vi "VisionTargetRead.vi"(5 "RobotConfig":T1={"Motors"={"DriveLeftPrimary"={"CAN Address"=1, "Invert"=FALSE, "InvertSensor"=FALSE, "Unit Conversion Factor"=0.0, "Brake Mode"=enum."Override to Brake", "Reverse Limt Switch Mode"=enum."Normally Closed", "Forward Limt Swith Mode"=enum."Normally Closed"}, "DriveLeftSecondary1"={"CAN Address"=2, "Invert"=FALSE, "InvertSensor"=FALSE, "Unit Conversion Factor"=0.0, "Brake Mode"=enum."Override to Brake", "Reverse Limt Switch Mode"=enum."Normally Closed", "Forward Limt Swith Mode"=enum."Normally Closed"}, "DriveRightPrimary"={"CAN Address"=3, "Invert"=FALSE, "InvertSensor"=FALSE, "Unit Conversion Factor"=0.0, "Brake Mode"=enum."Override to Brake", "Reverse Limt Switch Mode"=enum."Normally Closed", "Forward Limt Swith Mode"=enum."Normally Closed"}, "DriveRightSecondary1"={"CAN Address"=4, "Invert"=FALSE, "InvertSensor"=FALSE, "Unit Conversion Factor"=0.0, "Brake Mode"=enum."Override to Brake", "Reverse Limt Switch Mode"=enum."Normally Closed", "Forward Limt Swith Mode"=enum."Normally Closed"}, "RightIntake"={"CAN Address"=8, "Invert"=FALSE, "InvertSensor"=FALSE, "Unit Conversion Factor"=0.0, "Brake Mode"=enum."Override to Brake", "Reverse Limt Switch Mode"=enum."Normally Closed", "Forward Limt Swith Mode"=enum."Normally Closed"}, "LeftIntake"={"CAN Address"=7, "Invert"=FALSE, "InvertSensor"=FALSE, "Unit Conversion Factor"=0.0, "Brake Mode"=enum."Override to Brake", "Reverse Limt Switch Mode"=enum."Normally Closed", "Forward Limt Swith Mode"=enum."Normally Closed"}, "ArmPivot"={"CAN Address"=5, "Invert"=FALSE, "InvertSensor"=FALSE, "Unit Conversion Factor"=0.0, "Brake Mode"=enum."Override to Brake", "Reverse Limt Switch Mode"=enum."Normally Closed", "Forward Limt Swith Mode"=enum."Normally Closed"}, "ArmExtend"={"CAN Address"=6, "Invert"=FALSE, "InvertSensor"=FALSE, "Unit Conversion Factor"=0.0, "Brake Mode"=enum."Override to Brake", "Reverse Limt Switch Mode"=enum."Normally Closed", "Forward Limt Swith Mode"=enum."Normally Closed"}, "ArmPivot2"={"CAN Address"=9, "Invert"=FALSE, "InvertSensor"=FALSE, "Unit Conversion Factor"=0.0, "Brake Mode"=enum."Override to Brake", "Reverse Limt Switch Mode"=enum."Normally Closed", "Forward Limt Swith Mode"=enum."Normally Closed"}, "Climber"={"CAN Address"=10, "Invert"=FALSE, "InvertSensor"=FALSE, "Unit Conversion Factor"=0.0, "Brake Mode"=enum."Override to Brake", "Reverse Limt Switch Mode"=enum."Disabled", "Forward Limt Swith Mode"=enum."Disabled"}}, "Sensors"={"IMU"={"Yaw Axis"=enum."Z", "SPI Bus"=enum."SPI MXP", "AHRS Algorithm"=enum."Complementary", "Calibration Time (s)"=3.0, "Calibrate On Open"=TRUE}, "LimitSwitch1"={"DIOChannel"=enum."DIO 0", "Active Low"=FALSE}, "LimitSwitch2"={"DIOChannel"=enum."DIO 1", "Active Low"=FALSE}, "BeamBreak"={"DIOChannel"=enum."DIO 2", "Active Low"=FALSE}, "JeVois"={"Baud Rate"=9600, "Parity"=0, "Data Bits"=8, "Stop Bits"=10, "Termination Char (0xA = '\\n' = LF)"=10, "Enable Termination Char? (T)"=TRUE, "Flow Control"=0, "Timeout Value (ms)"=5000, "Serial Port"=enum."Onboard RS-232"}}, "PID"={"ArmExtend"={"P"=0.0, "I"=0.0, "D"=0.0, "F"=0.0, "IZone"=0.0}, "ArmRotate"={"P"=0.0, "I"=0.0, "D"=0.0, "F"=0.0, "IZone"=0.0}, "Drive"={"P"=0.0, "I"=0.0, "D"=0.0, "F"=0.0, "IZone"=0.0}}, "Solenoids"={"ArmClaw"={"Forward Channel"=enum."Solenoid 0", "Invert"=FALSE, "Reverse Channel"=enum."Solenoid 0"}, "IntakeExtend"={"Forward Channel"=enum."Solenoid 1", "Invert"=FALSE, "Reverse Channel"=enum."Solenoid 0"}, "IntakeOpen"={"Forward Channel"=enum."Solenoid 2", "Invert"=FALSE, "Reverse Channel"=enum."Solenoid 0"}, " Shifter"={"Forward Channel"=enum."Solenoid 3", "Invert"=FALSE, "Reverse Channel"=enum."Solenoid 0"}}, "RobotDimensions "={"Length"=0.0, "Height"=0.0, "HeightOfBumpers"=0.0, "DistanceFromFrameEdgeToPyramid "=0.0, "HeightOfFrameToIntake"=0.0, "EdgeOfFrameToOrigin"=0.0}, "ArmHomePosition"={"Angle (rad)"=0.0, "Radius (in)"=0.0}} {"Sensors"."JeVois"."Flow Control" items=["None", "XON/XOFF", "RTS/CTS", "XON/XOFF & RTS/CTS", "DTR/DSR", "XON/XOFF & DTR/DSR"]; "Sensors"."JeVois"."Termination Char (0xA = '\\n' = LF)" format="%.0x"; "Sensors"."JeVois"."Stop Bits" items=["1.0"=10, "1.5"=15, "2.0"=20]; "Sensors"."JeVois"."Parity" items=["None", "Odd", "Even", "Mark", "Space"]}, 6 "JeVois Camera DevRef":T16) -> (0 "error out":errorcluster, 1 "Right Vision Target":T17, 2 "Left Vision Target":T17, 3 "JeVoisOut":T16, 4 "Power Cube":T17)   [LabVIEW 2017]
uses:
  TypeDefs/VisionTarget.ctl
  General/PathPlanning/TypeDefs/Point2D.ctl
  TypeDefs/VisionTargetType.ctl
  <vilib>/Rock Robotics/WPI/SerialPort/WPI_SerialPortRef.ctl
  TypeDefs/ConfigComponents/Config_Robot.ctl
  TypeDefs/ConfigComponents/Config_Motor.ctl
  <vilib>/Rock Robotics/WPI/ThirdParty/Phoenix-LabVIEW/Motor Controller/Controls/CTRE_Phoenix_MotorControl_NeutralMode.ctl
  <vilib>/Rock Robotics/WPI/ThirdParty/Phoenix-LabVIEW/Motor Controller/Controls/CTRE_Phoenix_MotorControl_LimitSwitchNormal.ctl
  TypeDefs/ConfigComponents/Config_IMU.ctl
  <vilib>/Rock Robotics/SystemInterfaces/spilib/spi_bus.ctl
  TypeDefs/ConfigComponents/Config_DigitalIO.ctl
  <vilib>/Rock Robotics/SystemInterfaces/DIO/FPGA_DIOChannel.ctl
  TypeDefs/ConfigComponents/Config_SerialPort.ctl
  <vilib>/Rock Robotics/WPI/SerialPort/WPI_SerialPort.ctl
  TypeDefs/ConfigComponents/Config_PIDParams.ctl
  TypeDefs/ConfigComponents/Config_DoubleSolenoid.ctl
  <vilib>/Rock Robotics/WPI/Solenoid/WPI_SolenoidChannel.ctl
  TypeDefs/ConfigComponents/Config_Dimensions.ctl
  TypeDefs/ConfigComponents/Config_ArmHome.ctl
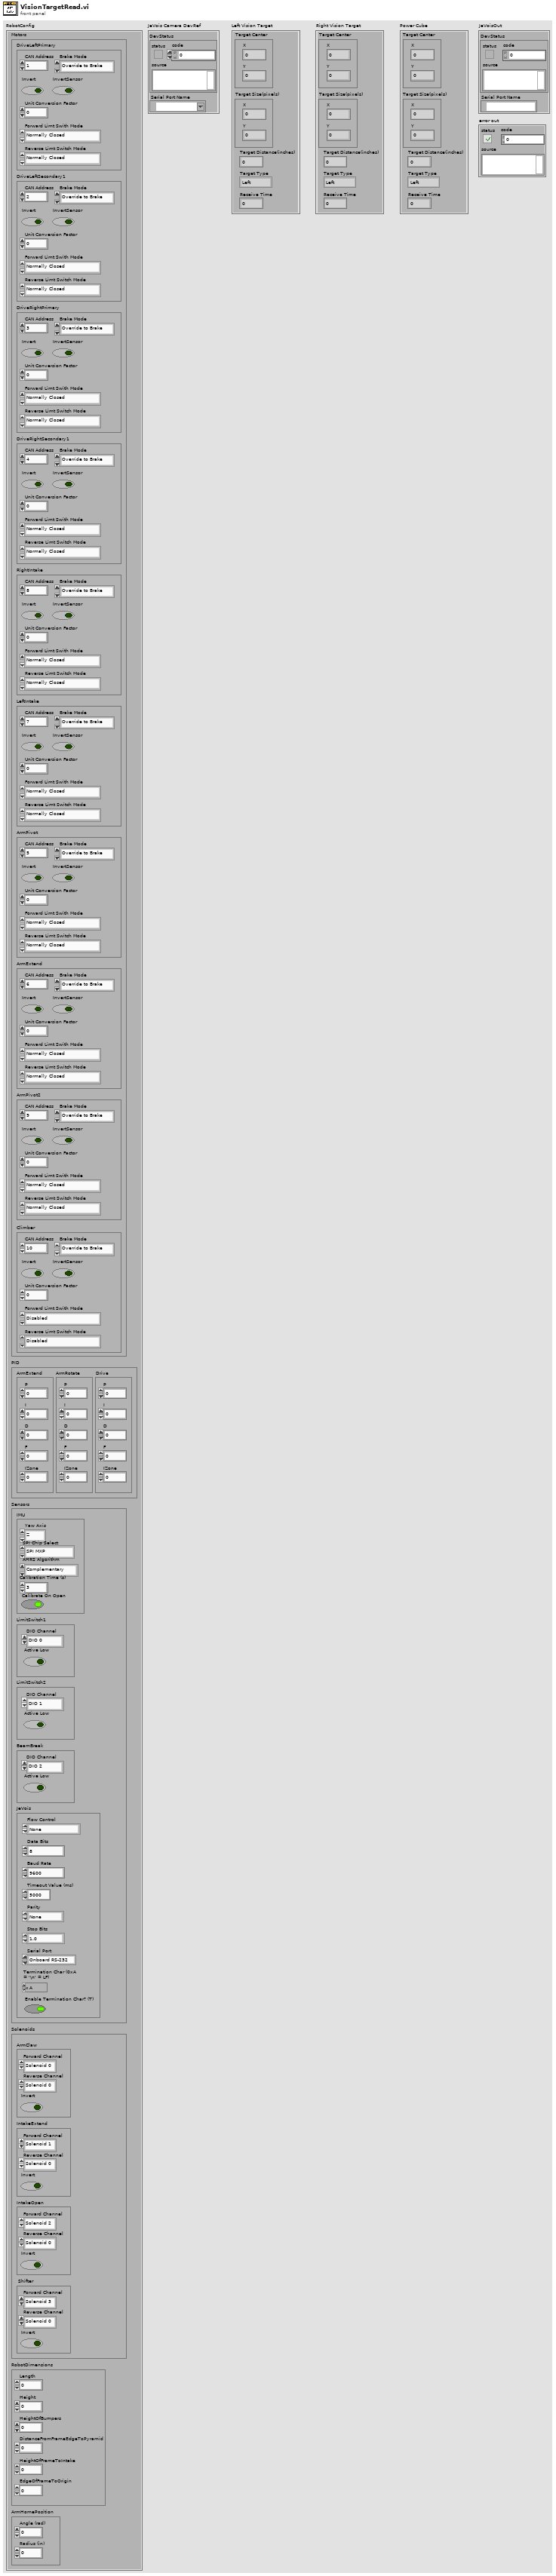
[diagram p1: front panel]
types:
  T1 = typedef "Config_Robot.ctl" = cluster{"Motors":cluster{"DriveLeftPrimary":T2, "DriveLeftSecondary1":T2, "DriveRightPrimary":T2, "DriveRightSecondary1":T2, "RightIntake":T2, "LeftIntake":T2, "ArmPivot":T2, "ArmExtend":T2, "ArmPivot2":T2, "Climber":T2}, "Sensors":cluster{"IMU":T5, "LimitSwitch1":T7, "LimitSwitch2":T7, "BeamBreak":T7, "JeVois":T9}, "PID":cluster{"ArmExtend":T11, "ArmRotate":T11, "Drive":T11}, "Solenoids":cluster{"ArmClaw":T12, "IntakeExtend":T12, "IntakeOpen":T12, " Shifter":T12}, "RobotDimensions ":T14, "ArmHomePosition":T15}
  T2 = typedef "Config_Motor.ctl" = cluster{"CAN Address":u8, "Invert":bool, "InvertSensor":bool, "Unit Conversion Factor":dbl, "Brake Mode":T3, "Reverse Limt Switch Mode":T4, "Forward Limt Swith Mode":T4}
  T3 = typedef "CTRE_Phoenix_MotorControl_NeutralMode.ctl" = enum8{"EEPROMSetting", "Override to Coast", "Override to Brake"}
  T4 = typedef "CTRE_Phoenix_MotorControl_LimitSwitchNormal.ctl" = enum16{"Normally Open", "Normally Closed", "Disabled"}
  T5 = typedef "Config_IMU.ctl" = cluster{"Yaw Axis":enum16{"X", "Y", "Z"}, "SPI Bus":T6, "AHRS Algorithm":enum16{"Complementary", "Madgwick"}, "Calibration Time (s)":dbl, "Calibrate On Open":bool}
  T6 = typedef "spi_bus.ctl" = enum16{"SPI On-Board, CS0", "SPI On-Board, CS1", "SPI On-Board, CS2", "SPI On-Board, CS3", "SPI MXP", "Invalid"}
  T7 = typedef "Config_DigitalIO.ctl" = cluster{"DIOChannel":T8, "Active Low":bool}
  T8 = typedef "FPGA_DIOChannel.ctl" = enum8{"DIO 0", "DIO 1", "DIO 2", "DIO 3", "DIO 4", "DIO 5", "DIO 6", "DIO 7", "DIO 8", "DIO 9", "DIO MXP 0", "DIO MXP 1", "DIO MXP 2", "DIO MXP 3", "DIO MXP 4", "DIO MXP 5", "DIO MXP 6", "DIO MXP 7", "DIO MXP 8", "DIO MXP 9", "DIO MXP 10", "DIO MXP 11", "DIO MXP 12", "DIO MXP 13", "DIO MXP 14", "DIO MXP 15", "SPI Port CS1", "SPI Port CS2", "SPI Port CS3", "SPI Port MISO", "SPI Port MOSI", "Invalid"}
  T9 = typedef "Config_SerialPort.ctl" = cluster{"Baud Rate":u32, "Parity":u16, "Data Bits":u16, "Stop Bits":u16, "Termination Char (0xA = '\\n' = LF)":u8, "Enable Termination Char? (T)":bool, "Flow Control":u16, "Timeout Value (ms)":u32, "Serial Port":T10}
  T10 = typedef "WPI_SerialPort.ctl" = enum16{"Onboard RS-232", "MXP TTL", "USB 1", "USB 2"}
  T11 = typedef "Config_PIDParams.ctl" = cluster{"P":dbl, "I":dbl, "D":dbl, "F":dbl, "IZone":dbl}
  T12 = typedef "Config_DoubleSolenoid.ctl" = cluster{"Forward Channel":T13, "Invert":bool, "Reverse Channel":T13}
  T13 = typedef "WPI_SolenoidChannel.ctl" = enum8{"Solenoid 0", "Solenoid 1", "Solenoid 2", "Solenoid 3", "Solenoid 4", "Solenoid 5", "Solenoid 6", "Solenoid 7", "Invalid"}
  T14 = typedef "Config_Dimensions.ctl" = cluster{"Length":dbl, "Height":dbl, "HeightOfBumpers":dbl, "DistanceFromFrameEdgeToPyramid ":dbl, "HeightOfFrameToIntake":dbl, "EdgeOfFrameToOrigin":dbl}
  T15 = typedef "Config_ArmHome.ctl" = cluster{"Angle (rad)":dbl, "Radius (in)":dbl}
  T16 = typedef "WPI_SerialPortRef.ctl" = cluster{"DevStatus":errorcluster, "Serial Port Name":refnum<visa-resource-name>}
  T17 = typedef "VisionTarget.ctl" = cluster{"Target Center":T18, "Target Size(pixels)":T18, "Target Distance(inches)":dbl, "Target Type":T19, "Receive Time":u32}
  T18 = typedef "Point2D.ctl" = cluster{"X":dbl, "Y":dbl}
  T19 = typedef "VisionTargetType.ctl" = enum16{"Left", "Right", "Cube", "Unknown"}
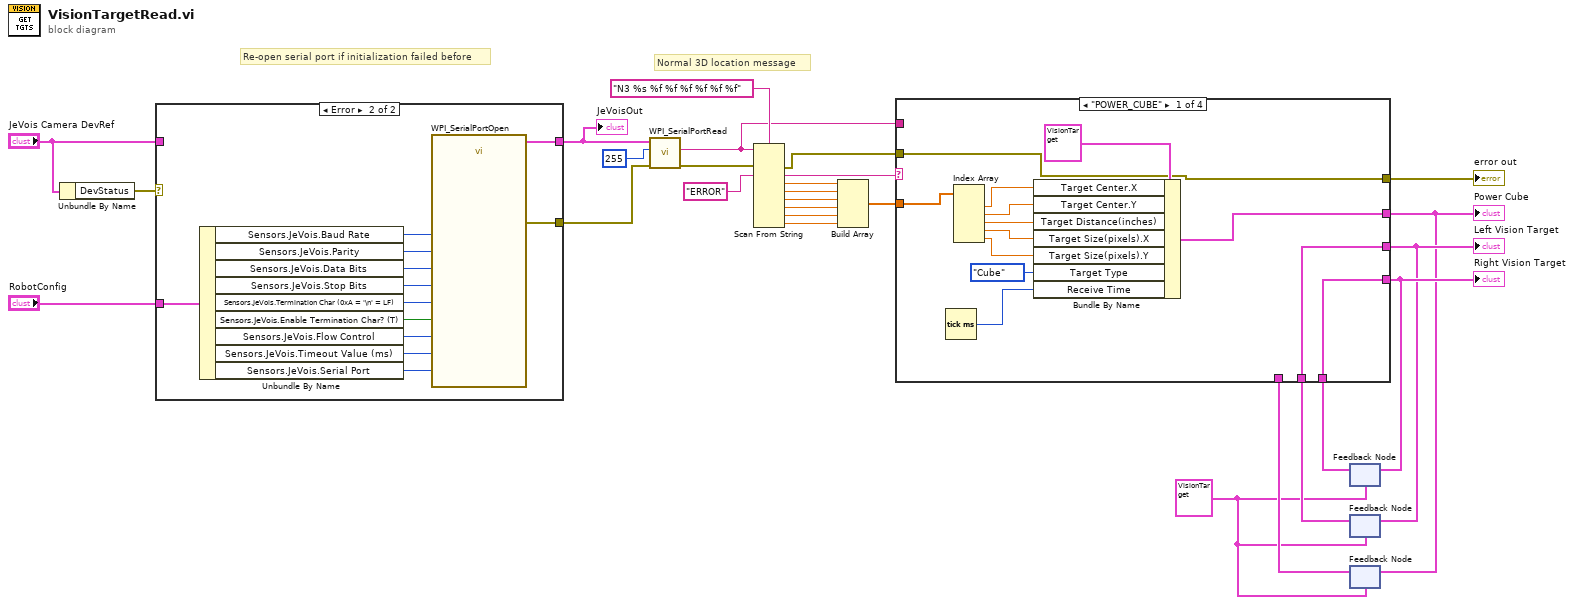
[diagram p0: block diagram]
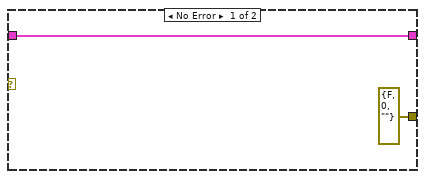
[diagram p2: hidden frame]
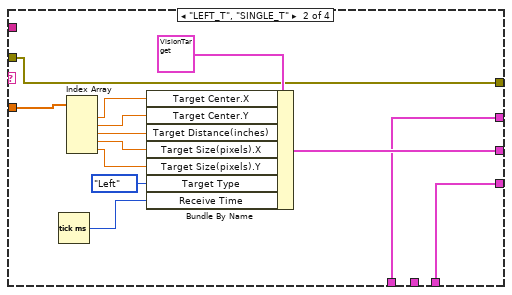
[diagram p3: hidden frame]
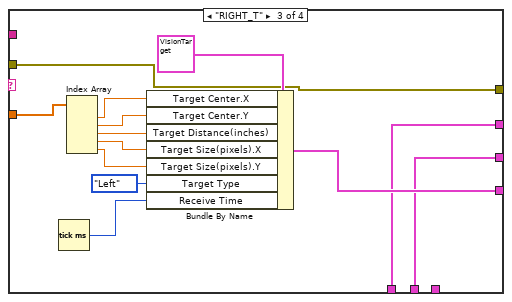
[diagram p4: hidden frame]
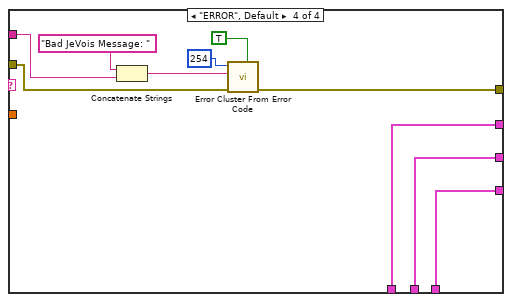
[diagram p5: hidden frame]
diagram:
  w8 = T17 {"Target Center"={"X"=0.0, "Y"=0.0}, "Target Size(pixels)"={"X"=0.0, "Y"=0.0}, "Target Distance(inches)"=0.0, "Target Type"=enum."Unknown", "Receive Time"=0} ("Left Vision Target")
  # "Re-open serial port if initialization failed before"
  # "Normal 3D location message"
  n1 = Unbundle By Name("JeVois Camera DevRef") -> ("DevStatus"=w5:errorcluster)
  n2 = case shown="Error" w5 {
    tunnel: [w29 w40] -> w3
    tunnel: "JeVois Camera DevRef" -> [w29 _]
    tunnel: [errorcluster {"status"=FALSE, "code"=0, "source"=""} ("error out") w41] -> w2
    tunnel: "RobotConfig" -> [_ w39]
    frame No Error {
    }
    frame Error {
      n3 = Unbundle By Name(w39) -> ("Sensors.JeVois.Baud Rate"=w38:u32, "Sensors.JeVois.Parity"=w37:u16, "Sensors.JeVois.Data Bits"=w36:u16, "Sensors.JeVois.Stop Bits"=w35:u16, "Sensors.JeVois.Termination Char (0xA = '\\n' = LF)"=w34:u8, "Sensors.JeVois.Enable Termination Char? (T)"=w33:bool, "Sensors.JeVois.Flow Control"=w32:u16, "Sensors.JeVois.Timeout Value (ms)"=w31:u32, "Sensors.JeVois.Serial Port"=w30:T10)
      n4 = call <vilib>:"WPI_SerialPortOpen.vi"("Baud Rate"=w38, "Timeout Value (ms)"=w31, "Termination Char (0xA = '\\n' = LF)"=w34, "Enable Termination Char? (T)"=w33, "Data Bits"=w36, "Parity"=w37, "Stop Bits"=w35, "Flow Control"=w32, "Serial Port"=w30) -> ("SerialPortRef"=w40:T16, "error out"=w41:errorcluster)  [unwired: 5 in]
    }
  }
  "JeVoisOut" <- w3
  n5 = call <vilib>:"WPI_SerialPortRead.vi"("error in (no error)"=w2, "Num Bytes to Read"=u32 255, "SerialPortRef"=w3) -> ("error out"=w7:errorcluster, "Buffer"=w23:string)  [unwired: 6 in, 1 out]
  n6 = Scan From String(format string="N3 %s %f %f %f %f %f %f", input string=w23, error in=w7, default 1="ERROR" ("default value 1")) -> (error out=w6:errorcluster, output 1=w24:string, output 2=w22:dbl, output 3=w21:dbl, output 4=w20:dbl, output 5=w19:dbl, output 6=w18:dbl, output 7=w17:dbl)  [unwired: 7 in, 2 out]
  n7 = Build Array(w22, w21, w20, w19, w18, w17) -> (w16:dbl[])
  n8 = feedback #1(w8) -> (w14:T17)
  n9 = feedback #2(w8) -> (w13:T17)
  n10 = feedback #3(w8) -> (w12:T17)
  n11 = case shown="\"POWER_CUBE\"" w24 {
    tunnel: w23 -> [_ _ _ w84]
    tunnel: w16 -> [w51 w64 w77 _]
    tunnel: [w45 w56 w69 w90] -> w10
    tunnel: [w43 w58 w70 w89] -> w11
    tunnel: [w44 w57 w71 w88] -> w15
    tunnel: w14 -> [w44 w57 _ w88]
    tunnel: w13 -> [w43 _ w70 w89]
    tunnel: w12 -> [_ w56 w69 w90]
    tunnel: [w42 w55 w68 w83] -> w9
    tunnel: w6 -> [w42 w55 w68 w82]
    frame "POWER_CUBE" {
      n12 = Tick Count (ms)() -> (millisecond timer value=w53:u32)
      n13 = Index Array(array=w51) -> (element #1=w50:dbl, element #2=w49:dbl, element #3=w48:dbl, element #4=w47:dbl, element #5=w46:dbl)  [unwired: 5 in]
      n14 = Bundle By Name(cluster=T17 {"Target Center"={"X"=0.0, "Y"=0.0}, "Target Size(pixels)"={"X"=0.0, "Y"=0.0}, "Target Distance(inches)"=0.0, "Target Type"=enum."Left", "Receive Time"=0} ("Left Vision Target"), "Target Center.X"=w50, "Target Center.Y"=w49, "Target Distance(inches)"=w48, "Target Size(pixels).X"=w47, "Target Size(pixels).Y"=w46, "Target Type"=VisionTargetType."Cube", "Receive Time"=w53) -> (w45:T17)
    }
    frame "LEFT_T", "SINGLE_T" {
      n15 = Tick Count (ms)() -> (millisecond timer value=w66:u32)
      n16 = Index Array(array=w64) -> (element #1=w63:dbl, element #2=w62:dbl, element #3=w61:dbl, element #4=w60:dbl, element #5=w59:dbl)  [unwired: 5 in]
      n17 = Bundle By Name(cluster=T17 {"Target Center"={"X"=0.0, "Y"=0.0}, "Target Size(pixels)"={"X"=0.0, "Y"=0.0}, "Target Distance(inches)"=0.0, "Target Type"=enum."Left", "Receive Time"=0} ("Left Vision Target"), "Target Center.X"=w63, "Target Center.Y"=w62, "Target Distance(inches)"=w61, "Target Size(pixels).X"=w60, "Target Size(pixels).Y"=w59, "Target Type"=VisionTargetType."Left", "Receive Time"=w66) -> (w58:T17)
    }
    frame "RIGHT_T" {
      n18 = Tick Count (ms)() -> (millisecond timer value=w79:u32)
      n19 = Index Array(array=w77) -> (element #1=w76:dbl, element #2=w75:dbl, element #3=w74:dbl, element #4=w73:dbl, element #5=w72:dbl)  [unwired: 5 in]
      n20 = Bundle By Name(cluster=T17 {"Target Center"={"X"=0.0, "Y"=0.0}, "Target Size(pixels)"={"X"=0.0, "Y"=0.0}, "Target Distance(inches)"=0.0, "Target Type"=enum."Left", "Receive Time"=0} ("Left Vision Target"), "Target Center.X"=w76, "Target Center.Y"=w75, "Target Distance(inches)"=w74, "Target Size(pixels).X"=w73, "Target Size(pixels).Y"=w72, "Target Type"=VisionTargetType."Left", "Receive Time"=w79) -> (w71:T17)
    }
    frame "ERROR", Default {
      n21 = Concatenate Strings("Bad JeVois Message: " ("string"), w84) -> (w86:string)
      n22 = call <vilib>:"Error Cluster From Error Code.vi"("is warning? (False)"=TRUE, "error in (no error)"=w82, "error message (\"\")"=w86, "error code (0)"=254) -> ("error out"=w83:errorcluster)  [unwired: 5 in]
    }
  }
  "Left Vision Target" <- w11
  "Right Vision Target" <- w15
  "Power Cube" <- w10
  "error out" <- w9
  n23 = feedback-in #1(w15) -> ()
  n24 = feedback-in #2(w11) -> ()
  n25 = feedback-in #3(w10) -> ()
